vi "Pre Launch Init.vi"(11 "Configurator Actor:Configuration UI Actor in":refnum<class "Configuration UI Actor.lvclass">) -> (0 "error out":errorcluster, 3 "Configurator Actor:Configuration UI Actor out":refnum<class "Configuration UI Actor.lvclass">)   [LabVIEW 2023, in "Configuration UI Actor.lvlib" / "Configuration UI Actor.lvclass"]
doc: "(<B>Filename</B>: Actor Framework.lvlib:Actor.lvclass:Pre Launch Init.vi)\n\nDefines behavior that occurs after the Launch Nested Actor method is invoked but before the actor's Actor Core method begins running.\n\nBy default, this method does nothing. A descendant class may override it to define behavior."
uses:
  Configuration UI Actor.lvclass
  Configuration UI Actor.lvclass/Configuration UI Actor.ctl
  CFG Provider/IProvide Configurations/IProvide Configurations.lvclass
  <vilib>/MGI/Panel Manager/Panel Actor/Panel Actor/Panel Actor.lvclass
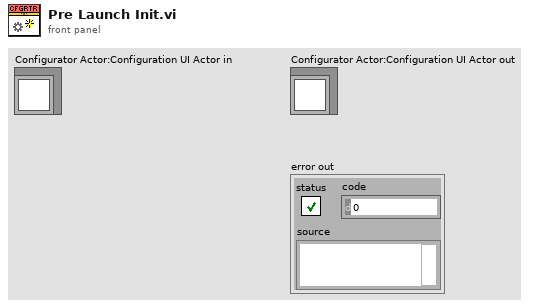
[diagram p1: front panel]
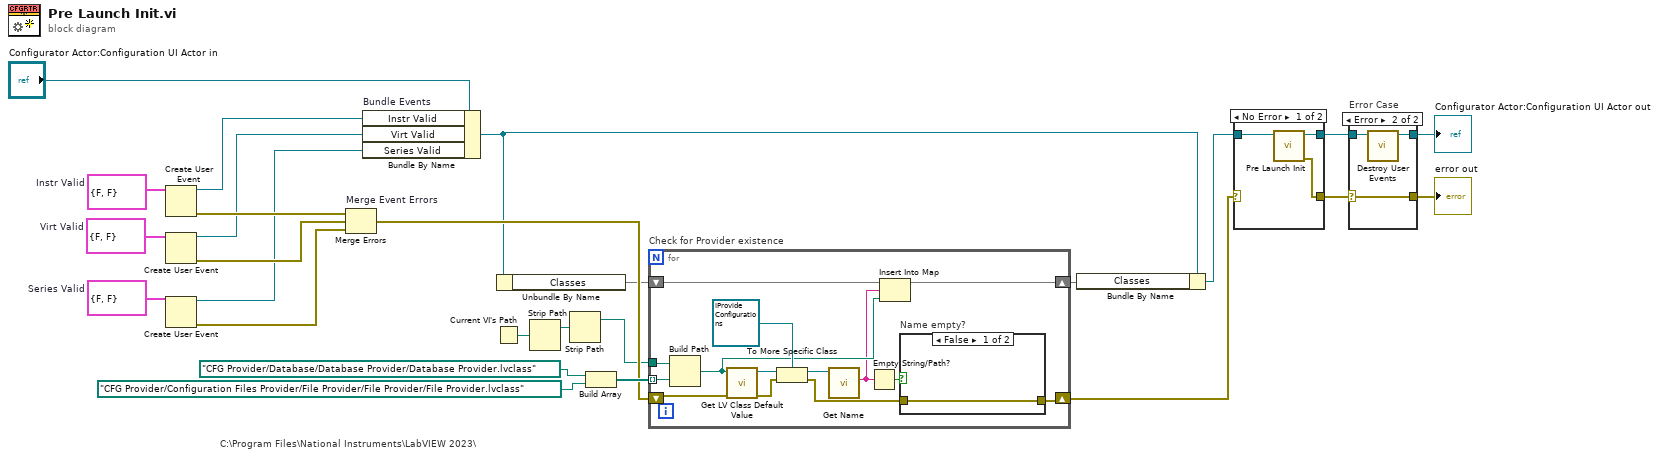
[diagram p0: block diagram]
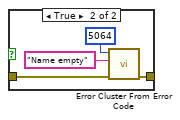
[diagram p2: hidden frame]
diagram:
  w15 = cluster{"JSON":bool, "CFG":bool} {"JSON"=FALSE, "CFG"=FALSE}  # Series Valid
  w18 = cluster{"JSON":bool, "CFG":bool} {"JSON"=FALSE, "CFG"=FALSE}  # Virt Valid
  w21 = cluster{"JSON":bool, "CFG":bool} {"JSON"=FALSE, "CFG"=FALSE}  # Instr Valid
  # "C:\\Program Files\\National Instruments\\LabVIEW 2023\\"
  n1 = Create User Event(user event datatype=w21) -> (user event=w20:refnum<user-event>, error out=w19:errorcluster)  [unwired: 1 in]
  n2 = Create User Event(user event datatype=w18) -> (user event=w17:refnum<user-event>, error out=w16:errorcluster)  [unwired: 1 in]
  n3 = Create User Event(user event datatype=w15) -> (user event=w13:refnum<user-event>, error out=w14:errorcluster)  [unwired: 1 in]
  n4 = Merge Errors "Merge Event Errors"(w19, w16, w14) -> (w8:errorcluster)
  n5 = Bundle By Name "Bundle Events"(cluster="Configurator Actor:Configuration UI Actor in", "Instr Valid"=w20, "Virt Valid"=w17, "Series Valid"=w13) -> (w7:refnum<class "Configuration UI Actor.lvclass">)
  n6 = Current VI's Path() -> (path=w3:path)
  n7 = Unbundle By Name(w7) -> ("Classes"=w6:map{string, path})
  n8 = Strip Path(path=w3) -> (stripped path=w2:path)  [unwired: 1 out]
  n9 = Strip Path(path=w2) -> (stripped path=w1:path)  [unwired: 1 out]
  n10 = Build Array(path "CFG Provider/Database/Database Provider/Database Provider.lvclass" ("name or relative path"), path "CFG Provider/Configuration Files Provider/File Provider/File Provider/File Provider.lvclass") -> (w10:path[])
  n11 = for "Check for Provider existence" {
    tunnel: w1 -> [w40]
    tunnel: w10 -> [w39] mode=indexing
    shift-right: [w27] -> w4
    shift-left: w8 -> [w35]
    shift-right: [w31] -> w5
    shift-left: w6 -> [w33]
    n12 = Build Path(base path=w40, name or relative path=w39) -> (appended path=w32:path)
    n13 = call <vilib>:"Get LV Class Default Value.vi"("error in (no error)"=w35, "class path"=w32) -> ("error out"=w36:errorcluster, "object"=w37:refnum<class>)  [unwired: 8 in]
    n14 = To More Specific Class(target class=refnum<class "IProvide Configurations.lvclass"> refnum ("IProvide Configurations.lvclass"), reference=w37, error in=w36) -> (specific class reference=w34:refnum<class "IProvide Configurations.lvclass">, error out=w28:errorcluster)
    n15 = call-dynamic "Get Name.vi"("IProvide Configurations in"=w34) -> ("Name"=w30:string)  [unwired: 9 in, 1 out]
    n16 = Empty String/Path?(string/path=w30) -> (empty?=w29:bool)
    n17 = Insert Into Map(map in=w33, key=w30, value=w32) -> (map out=w31:map{string, path})  [unwired: 2 out]
    n18 = case "Name empty?" shown="False" w29 {
      tunnel: w28 -> [w41 w45]
      tunnel: [w41 w44] -> w27
      frame False {
      }
      frame True {
        n19 = call <vilib>:"Error Cluster From Error Code.vi"("error in (no error)"=w45, "error message (\"\")"="Name empty" ("error message (\"\")"), "error code (0)"=5064) -> ("error out"=w44:errorcluster)  [unwired: 6 in]
      }
    }
  }
  n20 = Bundle By Name(cluster=w7, "Classes"=w5) -> (w9:refnum<class "Configuration UI Actor.lvclass">)
  n21 = case shown="No Error" w4 {
    selector: w4 -> [_ w50]
    tunnel: [w48 w49] -> w23
    tunnel: w9 -> [w47 w49]
    tunnel: [w46 w50] -> w22
    frame No Error {
      n22 = call-parent "Pre Launch Init.vi"("Panel Actor in"=w47) -> ("error out"=w46:errorcluster, "Panel Actor out"=w48:refnum<class "Configuration UI Actor.lvclass">)  [unwired: 9 in]
    }
    frame Error {
    }
  }
  n23 = case "Error Case" shown="Error" w22 {
    selector: w22 -> [w51 w55]
    tunnel: w23 -> [w52 w54]
    tunnel: [w52 w53] -> w25
    tunnel: [w51 w55] -> w24
    frame No Error {
    }
    frame Error {
      n24 = call "Destroy User Events.vi"("Configurator Actor:Configuration UI Actor in"=w54) -> ("Configurator Actor:Configuration UI Actor out"=w53:refnum<class "Configuration UI Actor.lvclass">)  [unwired: 10 in]
    }
  }
  "error out" <- w24
  "Configurator Actor:Configuration UI Actor out" <- w25
